vi "read_classes.vi"(8 "error in (no error)":errorcluster, 11 "SGDClassifier in":refnum<class "SGDClassifier.lvclass">) -> (0 "error out":errorcluster, 2 "classes":dbl[](array[numeric]), 3 "SGDClassifier out":refnum<class "SGDClassifier.lvclass">)   [LabVIEW 2020, in "SGDClassifier.lvclass"]
uses:
  SGDClassifier.lvclass
  SGDClassifier.lvclass/SGDClassifier.ctl
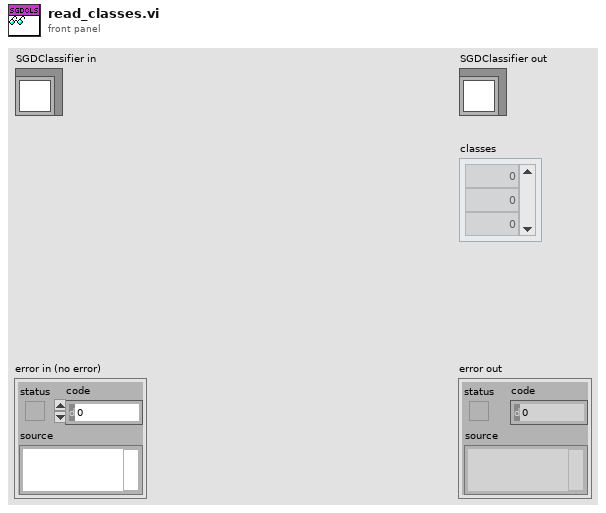
[diagram p1: front panel]
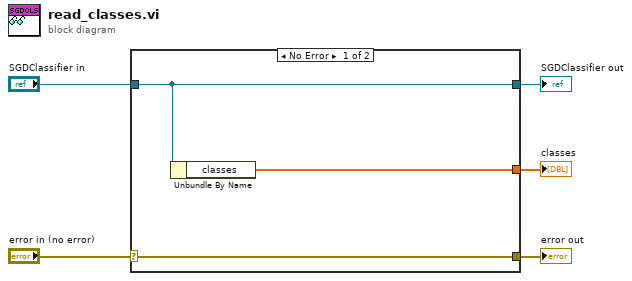
[diagram p0: block diagram]
diagram:
  n1 = case shown="No Error" "error in (no error)" {
    selector: "error in (no error)" -> [w8 w9]
    tunnel: [w8 w9] -> w4
    tunnel: [w7 w10] -> w2
    tunnel: "SGDClassifier in" -> [w7 w10]
    tunnel: [w6 _] -> w1
    frame No Error {
      n2 = Unbundle By Name(w7) -> ("classes"=w6:dbl[])
    }
    frame Error {
    }
  }
  "error out" <- w4
  "SGDClassifier out" <- w2
  "classes" <- w1
